vi "Read Configuration File.vi"(8 "error in (no error)":errorcluster, 11 "Instrument.OxfordVRM in":refnum<class "Instrument.OxfordVRM.lvclass">) -> (0 "error out":errorcluster, 3 "Instrument.OxfordVRM out":refnum<class "Instrument.OxfordVRM.lvclass">)   [LabVIEW 2019, in "Instrument.OxfordVRM.lvclass"]
uses:
  Instrument.OxfordVRM.lvclass
  C:/Program Files (x86)/National Instruments/LabVIEW 2019/user.lib/LevyLab/Instrument Framework/Instrument/Instrument.lvclass
  <userlib>/LevyLab/Instrument Framework/Instrument/Instrument.lvclass/Instrument.ctl
  <userlib>/LevyLab/Configuration/Configuration.lvclass/Configuration.ctl
  Instrument.OxfordVRM.lvclass/Instrument.OxfordVRM.ctl
  <userlib>/LevyLab/Configuration/Write Section.vi
  <userlib>/LevyLab/Instrument Framework/Instrument/Instrument.lvclass
  C:/Program Files (x86)/National Instruments/LabVIEW 2019/vi.lib/JKI/JKI SMO/SMO/SMO.lvclass
  <vilib>/JKI/JKI SMO/SMO/Protected/ThisLevelClassName.vi
  <userlib>/LevyLab/Instrument Framework/Instrument Types/Cryostat/Instrument.Cryostat.lvclass
  <userlib>/LevyLab/Configuration/Configuration.lvclass
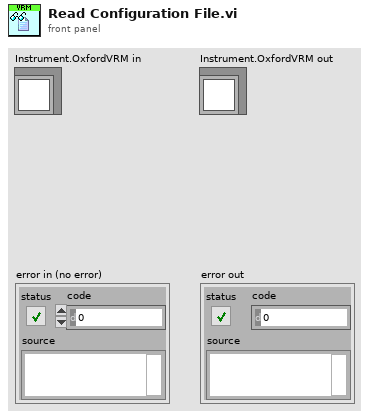
[diagram p1: front panel]
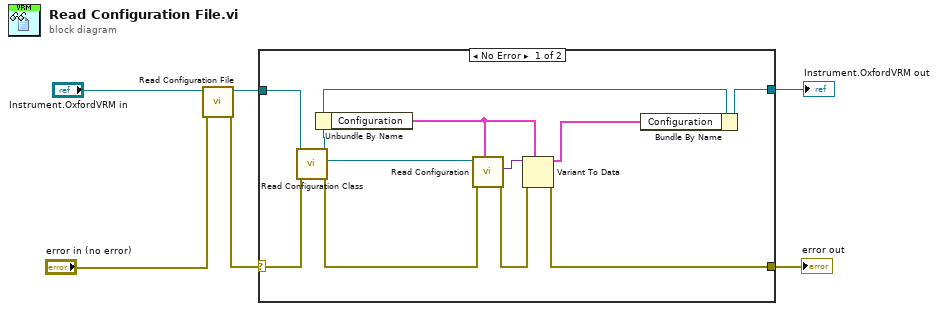
[diagram p0: block diagram]
diagram:
  n1 = call-parent "Read Configuration File.vi"("error in (no error)"="error in (no error)", "Instrument in"="Instrument.OxfordVRM in") -> ("error out"=w5:errorcluster, "Instrument out"=w2:refnum<class "Instrument.OxfordVRM.lvclass">)  [unwired: 8 in]
  n2 = case shown="No Error" w5 {
    selector: w5 -> [w14 w19]
    tunnel: [w13 w19] -> w3
    tunnel: [w17 w18] -> w1
    tunnel: w2 -> [w16 w18]
    frame No Error {
      n3 = call <userlib>:"Read Configuration Class.vi"("error in (no error)"=w14, "Instrument in"=w16) -> ("error out"=w11:errorcluster, "Configuration"=w10:refnum<class "Configuration.lvclass">, "Instrument out"=w15:refnum<class "Instrument.OxfordVRM.lvclass">)  [unwired: 7 in]
      n4 = Unbundle By Name(w15) -> ("Configuration"=w12:cluster{"IPS Address":string})
      n5 = call <userlib>:"Read Configuration.vi"("INI Fomatted Cluster Type"=w12, "error in (no error)"=w11, "Configuration in"=w10) -> ("error out"=w8:errorcluster, "Configuration"=w9:variant)  [unwired: 6 in, 1 out]
      n6 = Variant To Data(error in=w8, type=w12, Variant=w9) -> (data=w7:cluster{"IPS Address":string}, error out=w13:errorcluster)
      n7 = Bundle By Name(cluster=w15, "Configuration"=w7) -> (w17:refnum<class "Instrument.OxfordVRM.lvclass">)
    }
    frame Error {
    }
  }
  "Instrument.OxfordVRM out" <- w1
  "error out" <- w3
